vi "View-scan-file.vi"(8 "error in (no error)":errorcluster, 11 "Object ref in":T1) -> (0 "error out":errorcluster, 3 "Object ref out":T1)   [LabVIEW 2013, in "MaterialCharacterization.lvlib" / "MC-Main.lvclass"]
uses:
  MC-Main.lvclass
  Object-reference.ctl
  MC-Main.lvclass/MC-Main.ctl
  Read Scan file path.vi
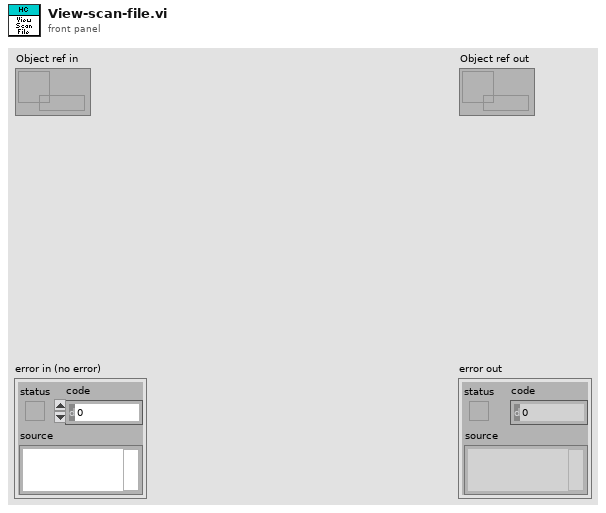
[diagram p1: front panel]
types:
  T1 = typedef "MaterialCharacterization.lvlib/MC-Main.lvclass/Object-reference.ctl" = refnum<data-value>
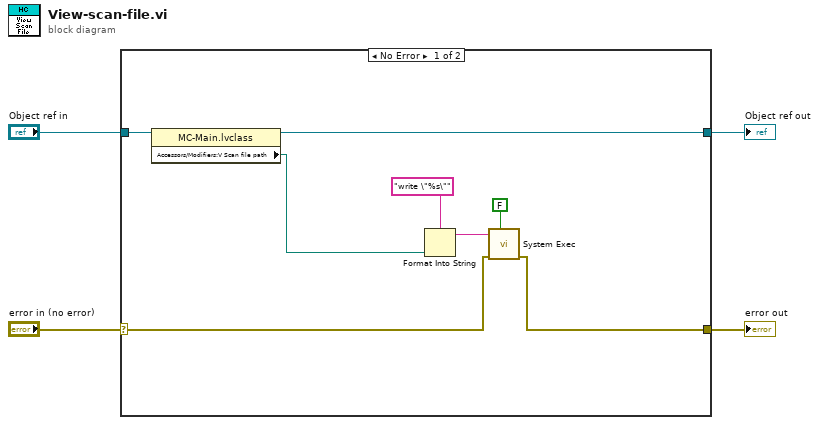
[diagram p0: block diagram]
diagram:
  n1 = case shown="No Error" "error in (no error)" {
    selector: "error in (no error)" -> [w6 w14]
    tunnel: [w5 w14] -> w3
    tunnel: [w8 w13] -> w1
    tunnel: "Object ref in" -> [w12 w13]
    frame No Error {
      n2 = property class="MC-Main.lvclass"(reference=w12) -> (reference out=w8:T1, "Accessors/Modifiers:V Scan file path"=w7:path)  [unwired: 1 in, 1 out]
      n3 = Format Into String(format string="write \"%s\"", w7) -> (resulting string=w9:string)  [unwired: 2 in, 1 out]
      n4 = call <vilib>:"System Exec.vi"("wait until completion? (T)"=FALSE, "error in (no error)"=w6, "command line"=w9) -> ("error out"=w5:errorcluster)  [unwired: 5 in, 3 out]
    }
    frame Error {
    }
  }
  "error out" <- w3
  "Object ref out" <- w1
